vi "Analog IO Message - Continuous Pin Report.vi"(8 "error in (no error)":errorcluster, 9 "Enable Continuous Reporting?":bool, 10 "Pin Index":u8) -> (0 "error out":errorcluster, 1 "Pin Value":u16, 2 "Pin Index Out":u8 format="%.0x")   [LabVIEW 2020, in "FirmataClient.lvlib"]
doc: "Allows requesting the state of a analog pin."
uses:
  FirmataClient.lvlib
panel:
  in  "Queue Name":string="firmata-serial-communication"
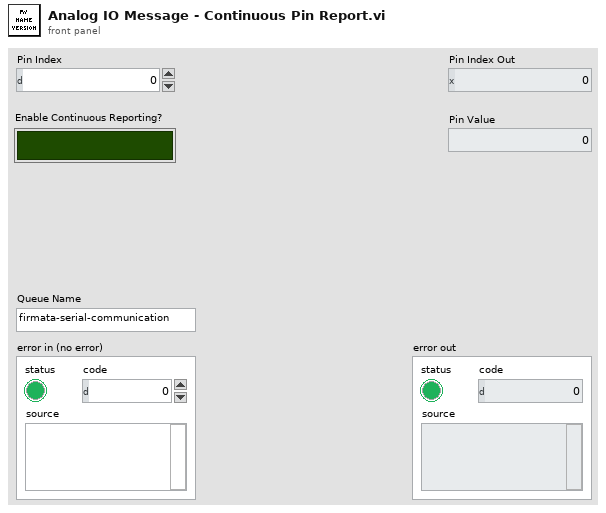
[diagram p1: front panel]
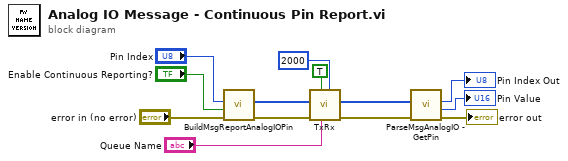
[diagram p0: block diagram]
diagram:
  n1 = call "BuildMsgReportAnalogIOPin.vi"("error in"="error in (no error)", "Enable Continuous Reporting?"="Enable Continuous Reporting?", "Pin Index"="Pin Index") -> ("error out"=w3:errorcluster, "AnalogIOMessage"=w4:u8[])  [unwired: 5 in, 2 out]
  n2 = call "TxRx.vi"("Reply Timeout Ms"=2000, "Queue Name"="Queue Name", "Wait For Reply?"=TRUE, "error in"=w3, "Message"=w4) -> ("error out"=w2:errorcluster, "Reply"=w1:u8[])  [unwired: 5 in]
  n3 = call "ParseMsgAnalogIO - GetPin.vi"("error in"=w2, "Message"=w1) -> ("error out"=→"error out":errorcluster, "Pin Value"=→"Pin Value":u16, "Pin Index"=→"Pin Index Out":u8)  [unwired: 7 in]
